vi "20211015_04.vi"() -> ()   [LabVIEW 2019]
panel:
  out "Result string":string
  in  "People":i32
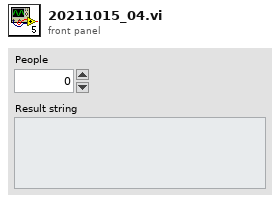
[diagram p1: front panel]
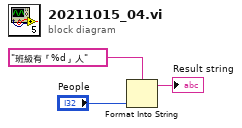
[diagram p0: block diagram]
diagram:
  n1 = Format Into String(format string="班級有「%d」人", "People") -> (resulting string=→"Result string":string)  [unwired: 2 in, 1 out]
